vi "Genetic Algorithm Test.vi"() -> ()   [LabVIEW 2013]
panel:
  out "Execution Time":i64
  out "Hamming Distance":u32
  out "Winner Display":T1(plugin-control)
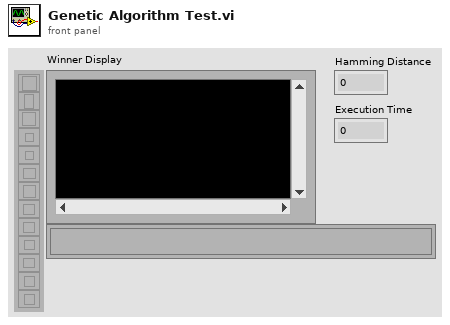
[diagram p1: front panel]
types:
  T1 = typedef "IMAQ Image.ctl" = refnum<image>
  T2 = typedef "Image Type" = u32
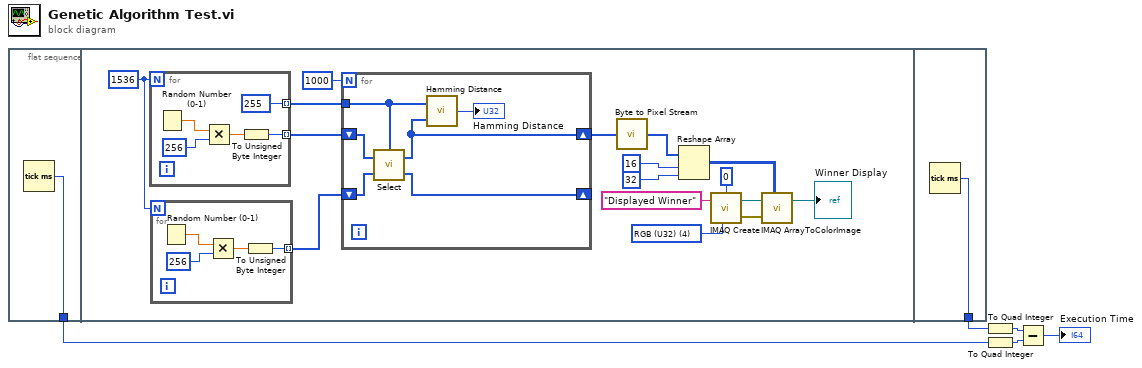
[diagram p0: block diagram]
diagram:
  n1 = flat-sequence {
    tunnel: [w6] -> w1
    tunnel: [w38] -> w2
    frame #0 {
      n2 = Tick Count (ms)() -> (millisecond timer value=w6:u32)
    }
    frame #1 {
      w7 = T2 4 items=["Grayscale (U8)", "Grayscale (I16)", "Grayscale (SGL)", "Complex (CSG)", "RGB (U32)", "HSL (U32)", "RGB (U64)", "Grayscale (U16)"] ("Image Type")
      w21 = 1536
      n3 = for {
        N: w21 -> [_]
        tunnel: [w34] -> w8 mode=indexing
        tunnel: [u8 255] -> w10 mode=indexing
        n4 = Random Number (0-1)() -> (number: 0 to 1=w35:dbl)
        n5 = Multiply(x=w35, y=256) -> (x*y=w37:dbl)
        n6 = To Unsigned Byte Integer(number=w37) -> (unsigned 8bit integer=w34:u8)
      }
      n7 = for {
        N: w21 -> [_]
        tunnel: [w23] -> w22 mode=indexing
        n8 = Random Number (0-1)() -> (number: 0 to 1=w26:dbl)
        n9 = Multiply(x=w26, y=256) -> (x*y=w24:dbl)
        n10 = To Unsigned Byte Integer(number=w24) -> (unsigned 8bit integer=w23:u8)
      }
      n11 = for {
        N: 1000 -> [_]
        shift-right: [w28] -> w20
        shift-left: w8 -> [w32]
        shift-right: [w30] -> _
        shift-left: w22 -> [w31]
        tunnel: w10 -> [w29]
        n12 = call "Select.vi"("Father"=w31, "Mother"=w32, "Target"=w29) -> ("Runnerup"=w30:u8[], "Winner"=w28:u8[])
        n13 = call "Hamming Distance.vi"("LED 2"=w28, "LED 1"=w29) -> ("Hamming Distance"=→"Hamming Distance":u32)
      }
      n14 = call "Byte to Pixel Stream.vi"("RGB Byte Stream"=w20) -> ("Pixel Stream"=w19:u32[])
      n15 = Reshape Array ("Reshape Array 2")(w19, 16 ("Constant 6"), 32 ("Constant 7")) -> (w14:u32[][])
      n16 = call "IMAQ Create"("Border Size"=0 ("Constant 9"), "Image Name"="Displayed Winner" ("Constant 8"), "Image Type"=w7) -> ("New Image"=w15:T1, "error out"=w16:errorcluster)  [unwired: 2 in]
      n17 = call "IMAQ ArrayToColorImage"("Image Pixels (U32)"=w14, "Image"=w15, "error in (no error)"=w16) -> ("Image Out"=→"Winner Display":T1)  [unwired: 2 in, 1 out]
    }
    frame #2 {
      n18 = Tick Count (ms)() -> (millisecond timer value=w38:u32)
    }
  }
  n19 = To Quad Integer(1:w2) -> (0:w4:i64)
  n20 = To Quad Integer(1:w1) -> (0:w3:i64)
  n21 = Subtract(x=w4, y=w3) -> (x-y=→"Execution Time":i64)
